vi "mxwScript_API_Option_SetStartDiagram(Location).vi"(0 "options in":T2[](array[typedef]), 1 "Position":T1, 2 "ClassName":string, 3 "error in (no error)":errorcluster, 4 "Frame":u32) -> (7 "options out":T2[](array[typedef]), 10 "error out":errorcluster)   [LabVIEW 2020]
doc: "Sets the password so password protected VIs can be generated into."
uses:
  codeGenAPISupport.llb/cgAPI_mxwScript_OptionData.ctl
  <vilib>/Utility/miscctls.llb/LVPositionTypeDef.ctl
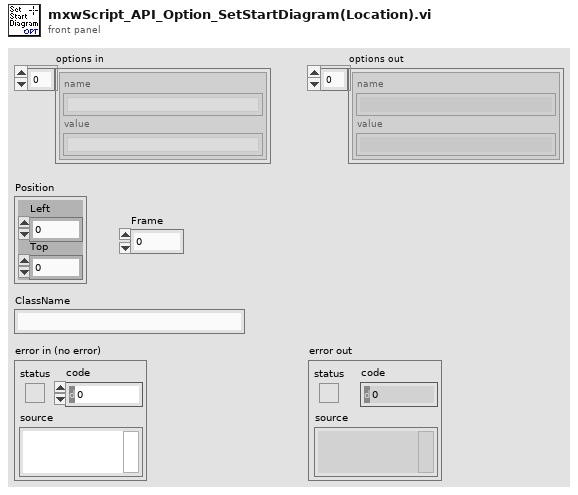
[diagram p1: front panel]
types:
  T1 = typedef "LVPositionTypeDef.ctl" = cluster{"Left":i32, "Top":i32}
  T2 = typedef "cgAPI_mxwScript_OptionData.ctl" = cluster{"name":string, "value":string}
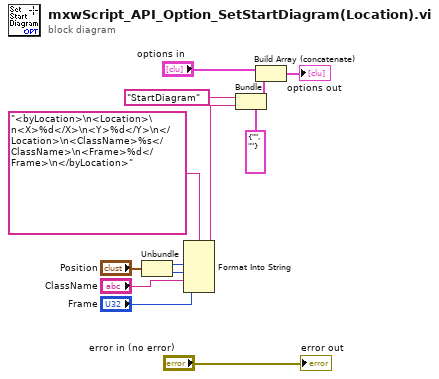
[diagram p0: block diagram]
diagram:
  n1 = Unbundle("Position") -> ("Left"=w5:i32, "Top"=w4:i32)
  n2 = Format Into String(format string="<byLocation>\n<Location>\n<X>%d</X>\n<Y>%d</Y>\n</Location>\n<ClassName>%s</ClassName>\n<Frame>%d</Frame>\n</byLocation>", w5, w4, "ClassName", "Frame") -> (resulting string=w1:string)  [unwired: 2 in, 1 out]
  n3 = Bundle(cluster=T2 {"name"="", "value"=""} ("optionData"), "name"="StartDiagram", "value"=w1) -> (w11:T2)
  n4 = Build Array (concatenate)("options in", w11) -> (→"options out":T2[])
  "error out" <- "error in (no error)"
